vi "Read Rate.vi"(8 "error in (no error)":errorcluster, 11 "TimingGrp in":refnum<class "TimingGrp.lvclass">) -> (0 "error out":errorcluster, 2 "Rate":dbl, 3 "TimingGrp out":refnum<class "TimingGrp.lvclass">)   [LabVIEW 2018, in "Configuration Grandmaster.lvlib" / "TimingGrp.lvclass"]
uses:
  TimingGrp.lvclass
  TimingGrp.lvclass/TimingGrp.ctl
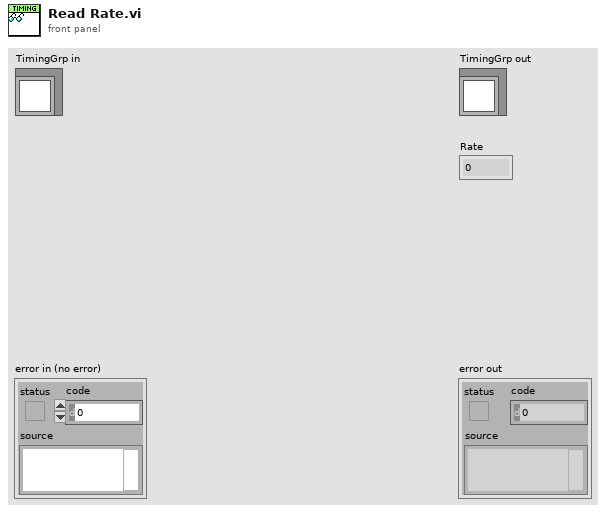
[diagram p1: front panel]
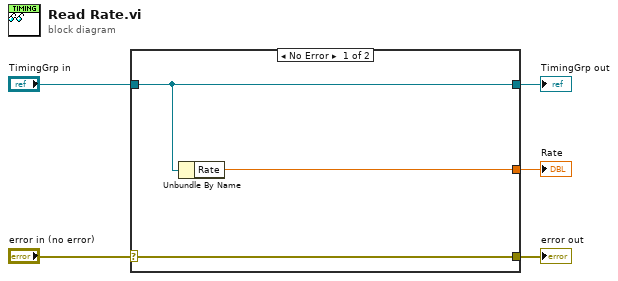
[diagram p0: block diagram]
diagram:
  n1 = case shown="No Error" "error in (no error)" {
    selector: "error in (no error)" -> [w8 w9]
    tunnel: [w8 w9] -> w4
    tunnel: [w7 w10] -> w2
    tunnel: "TimingGrp in" -> [w7 w10]
    tunnel: [w6 _] -> w1
    frame No Error {
      n2 = Unbundle By Name(w7) -> ("Rate"=w6:dbl)
    }
    frame Error {
    }
  }
  "error out" <- w4
  "TimingGrp out" <- w2
  "Rate" <- w1
